vi "Substitute the assigned name for Test.vi"(8 "error in":errorcluster, 10 "Project Name":string, 11 "Name to VI Map":map{string, refnum<vi>}(c390)) -> (0 "error out":errorcluster)   [LabVIEW 2023, in "Plugin Generator.lvlib"]
uses:
  Plugin Generator.lvlib
  <vilib>/Utility/traverseref.llb/TRef TravTarget.ctl
  <vilib>/Utility/traverseref.llb/VI Scripting - Traverse.lvlib
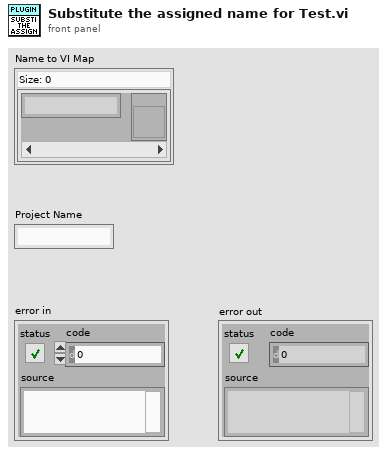
[diagram p1: front panel]
types:
  T1 = typedef "TRef TravTarget.ctl" = enum16{"FP", "BD", "Other"}
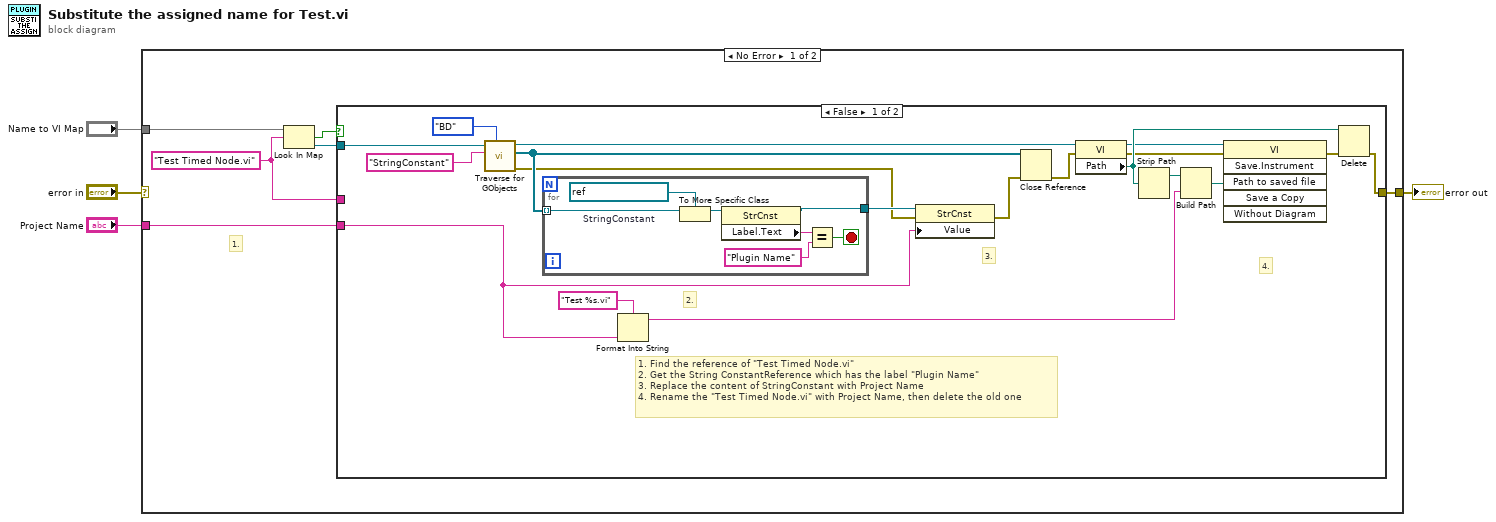
[diagram p0: block diagram]
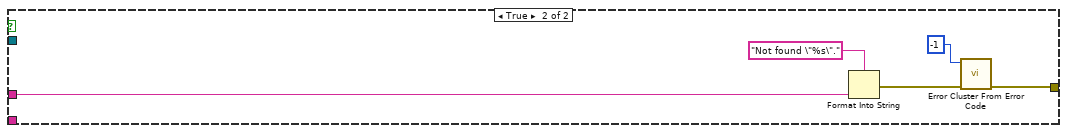
[diagram p2: hidden frame]
diagram:
  n1 = case shown="No Error" "error in" {
    selector: "error in" -> [_ w42]
    tunnel: [w10 w42] -> w4
    tunnel: "Project Name" -> [w9 _]
    tunnel: "Name to VI Map" -> [w8 _]
    frame No Error {
      w5 = "Test Timed Node.vi" ("String")
      # "1."
      n2 = Look In Map(map=w8, key=w5) -> (key not found?=w6:bool, value=w7:refnum<vi>)  [unwired: 1 in]
      n3 = case shown="False" w6 {
        tunnel: [w26 w41] -> w10
        tunnel: w9 -> [w12 _]
        tunnel: w7 -> [w11 _]
        tunnel: w5 -> [_ w37]
        frame False {
          # "4."
          # "3."
          # "2."
          # "1. Find the reference of \"Test Timed Node.vi\"\n2. Get the String ConstantReference which has the label \"Plugin Name\"\n3. Replace the content of StringConstant with Project Name\n4. Rename the \"Test Timed Node.vi\" with Project Name, then delete the old one"
          n4 = call <vilib>:"Traverse for GObjects.vi"("Traverse Target"=TRef_TravTarget."BD", "Class Name"="StringConstant", "VI Refnum"=w11) -> ("error out"=w14:errorcluster, "References"=w19:refnum<vi>[], "dup VI Refnum"=w15:refnum<vi>)  [unwired: 5 in, 1 out]
          n5 = for {
            tunnel: w19 -> [w36] mode=indexing
            tunnel: [w30] -> w18
            stop <- w31 stop-if-true
            w35 = refnum<vi> refnum  # StringConstant
            n6 = To More Specific Class(target class=w35, reference=w36) -> (specific class reference=w34:refnum<vi>)  [unwired: 1 in, 1 out]
            n7 = property class="StrCnst"(reference=w34) -> (reference out=w30:refnum<vi>, "Label.Text"=w33:string)  [unwired: 1 in, 1 out]
            n8 = Equal?(x=w33, y="Plugin Name") -> (x = y?=w31:bool)
          }
          n9 = Format Into String(format string="Test %s.vi", w12) -> (resulting string=w27:string)  [unwired: 2 in, 1 out]
          n10 = property class="StrCnst"(reference=w18, error in=w14, "Value"=w12) -> (error out=w20:errorcluster)  [unwired: 1 out]
          n11 = Close Reference(reference=w19, error in (no error)=w20) -> (error out=w13:errorcluster)
          n12 = property class="VI"(reference=w15, error in=w13) -> (reference out=w24:refnum<vi>, error out=w22:errorcluster, "Path"=w25:path)
          n13 = Strip Path(path=w25) -> (stripped path=w23:path)  [unwired: 1 out]
          n14 = Build Path(base path=w23, name or relative path=w27) -> (appended path=w28:path)
          n15 = invoke class="VI" method="Save.Instrument"(reference=w24, error in=w22, "Path to saved file"=w28) -> (error out=w21:errorcluster)  [unwired: 3 in, 5 out]
          n16 = Delete(path (use dialog)=w25, error in=w21) -> (error out=w26:errorcluster)  [unwired: 3 in, 2 out]
        }
        frame True {
          n17 = Format Into String(format string="Not found \"%s\"." ("error message (\"\")"), w37) -> (error out=w39:errorcluster)  [unwired: 2 in, 1 out]
          n18 = call <vilib>:"Error Cluster From Error Code.vi"("error in (no error)"=w39, "error code (0)"=-1) -> ("error out"=w41:errorcluster)  [unwired: 7 in]
        }
      }
    }
    frame Error {
    }
  }
  "error out" <- w4
